vi "dec string to i32 small.vi"(7 "String":string) -> (8 "number":i32)   [LabVIEW 2018]
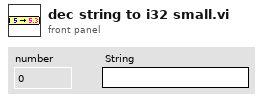
[diagram p1: front panel]
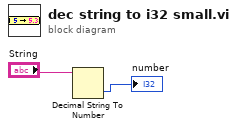
[diagram p0: block diagram]
diagram:
  n1 = Decimal String To Number(string="String") -> (number=→"number":i32)  [unwired: 2 in, 1 out]
